vi "crc16_dec.vi"(11 "Bit and crc16":i16[](array[numeric])) -> (3 "passed":bool)   [LabVIEW 2014]
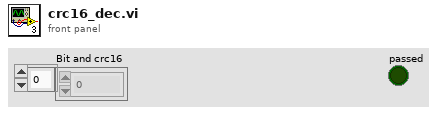
[diagram p1: front panel]
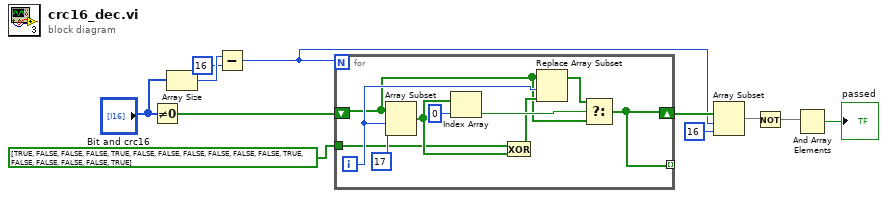
[diagram p0: block diagram]
diagram:
  n1 = Not Equal To 0?(x="Bit and crc16") -> (x != 0?=w8:bool[])
  n2 = Array Size(array="Bit and crc16") -> (size(s)=w10:i32)
  n3 = Subtract(x=w10, y=16) -> (x-y=w6:i32)
  n4 = for {
    N: w6 -> [_]
    shift-right: [w13] -> w7
    shift-left: w8 -> [w14]
    tunnel: [w13] -> _ mode=indexing
    tunnel: bool[] [TRUE, FALSE, FALSE, FALSE, TRUE, FALSE, FALSE, FALSE, FALSE, FALSE, FALSE, TRUE, FALSE, FALSE, FALSE, FALSE, TRUE] -> [w12]
    i -> [w17]
    n5 = Array Subset(array=w14, index=w17, length=17) -> (w19:bool[])
    n6 = Index Array(array=w19, index=0) -> (element=w18:bool)
    n7 = Exclusive Or(1:w19, 2:w12) -> (0:w16:bool[])
    n8 = Replace Array Subset(array=w14, new element=w16, index=w17) -> (w15:bool[])
    n9 = Select(t=w15, s=w18, f=w14) -> (s? t:f=w13:bool[])
  }
  n10 = Array Subset(array=w7, index=w6, length=16) -> (w4:bool[])
  n11 = Not(x=w4) -> (.not. x?=w3:bool[])
  n12 = And Array Elements(Boolean array=w3) -> (logical AND=→"passed":bool)
